vi "DriveStraight.vi"(6 "Reverse?":bool, 7 "Sensitivity":dbl, 8 "Range":dbl, 9 "Motor Speed":dbl, 10 "Target":dbl, 11 "Yaw":dbl) -> (0 "Right":dbl, 3 "Left":dbl)   [LabVIEW 2016]
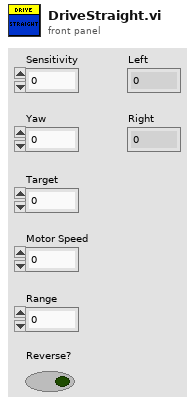
[diagram p1: front panel]
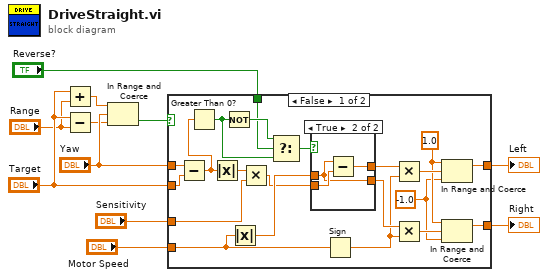
[diagram p0: block diagram]
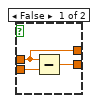
[diagram p2: hidden frame]
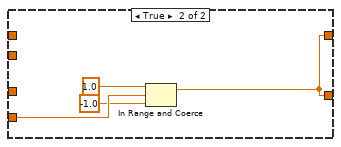
[diagram p3: hidden frame]
diagram:
  n1 = Add(x="Target", y="Range") -> (x+y=w5:dbl)
  n2 = Subtract(x="Target", y="Range") -> (x-y=w3:dbl)
  n3 = In Range and Coerce(upper limit=w5, x="Yaw", lower limit=w3) -> (In Range?=w8:bool)  [unwired: 1 out]
  n4 = case shown="False" w8 {
    tunnel: "Motor Speed" -> [w27 w42]
    tunnel: [w20 w39] -> w10
    tunnel: [w21 w39] -> w9
    tunnel: "Yaw" -> [w32 _]
    tunnel: "Sensitivity" -> [w28 _]
    tunnel: "Target" -> [w31 _]
    tunnel: "Reverse?" -> [w13 _]
    frame False {
      w22 = -1.0 ("lower limit")
      w24 = 1.0 ("upper limit")
      n5 = Subtract(x=w32, y=w31) -> (x-y=w30:dbl)
      n6 = Greater Than 0?(x=w30) -> (x > 0?=w14:bool)
      n7 = Absolute Value(x=w30) -> (abs(x)=w29:dbl)
      n8 = Not(x=w14) -> (.not. x?=w15:bool)
      n9 = Absolute Value(x=w27) -> (abs(x)=w17:dbl)
      n10 = Multiply(x=w29, y=w28) -> (x*y=w16:dbl)
      n11 = Select(t=w15, s=w13, f=w14) -> (s? t:f=w12:bool)
      n12 = case shown="True" w12 {
        tunnel: w17 -> [w34 w36]
        tunnel: w16 -> [w35 w37]
        tunnel: [w34 w38] -> w19
        tunnel: [w33 w36] -> w26
        frame False {
          n13 = Subtract(x=w34, y=w35) -> (x-y=w33:dbl)
        }
        frame True {
          n14 = Subtract(x=w36, y=w37) -> (x-y=w38:dbl)
        }
      }
      n15 = Sign(1:w27) -> (0:w18:dbl)
      n16 = Multiply(x=w19, y=w18) -> (x*y=w25:dbl)
      n17 = Multiply(x=w26, y=w18) -> (x*y=w23:dbl)
      n18 = In Range and Coerce(upper limit=w24, x=w25, lower limit=w22) -> (coerced(x)=w21:dbl)  [unwired: 1 out]
      n19 = In Range and Coerce(upper limit=w24, x=w23, lower limit=w22) -> (coerced(x)=w20:dbl)  [unwired: 1 out]
    }
    frame True {
      n20 = In Range and Coerce(upper limit=1.0, x=w42, lower limit=-1.0) -> (coerced(x)=w39:dbl)  [unwired: 1 out]
    }
  }
  "Left" <- w9
  "Right" <- w10
